vi "RGA Pressure Color ramp Set.vi"(8 "error in (no error)":errorcluster, 11 "reference":refnum<vi>) -> (0 "error out":errorcluster, 3 "reference out":refnum<vi>)   [LabVIEW 2018]
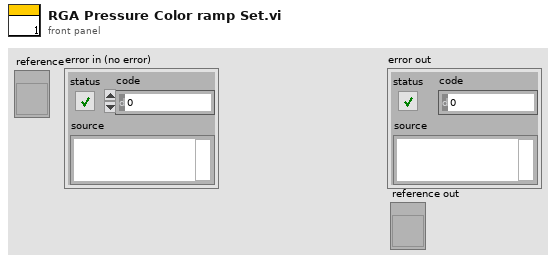
[diagram p1: front panel]
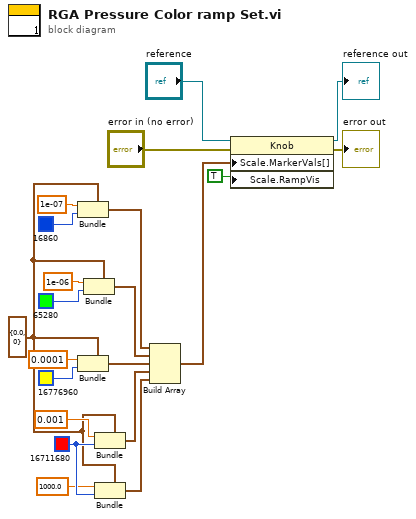
[diagram p0: block diagram]
diagram:
  w14 = u32 16711680 ("Color Box")
  w5 = cluster{dbl, u32} {0.0, 0}
  n1 = Bundle(cluster=w5, 1e-07, u32 16860 ("Color Box")) -> (w2:cluster{dbl, u32})
  n2 = Bundle(cluster=w5, 0.0001, u32 16776960 ("Color Box")) -> (w17:cluster{dbl, u32})
  n3 = Bundle(cluster=w5, 1e-06, u32 65280 ("Color Box")) -> (w1:cluster{dbl, u32})
  n4 = Bundle(cluster=w5, 0.001, w14) -> (w15:cluster{dbl, u32})
  n5 = Bundle(cluster=w5, 1000.0, w14) -> (w12:cluster{dbl, u32})
  n6 = Build Array(w2, w1, w17, w15, w12) -> (w10:cluster{dbl, u32}[])
  n7 = property class="Knob"(reference="reference", error in="error in (no error)", "Scale.MarkerVals[]"=w10, "Scale.RampVis"=TRUE ("Scale.Ramp Visible")) -> (reference out=→"reference out":refnum<vi>, error out=→"error out":errorcluster)
